vi "EventQueueCluster.vi"() -> ()   [LabVIEW 2017]
uses:
  EventQueueCluster.ctl
  EventMessage.ctl
panel:
  in  "EventQueueCluster":T1
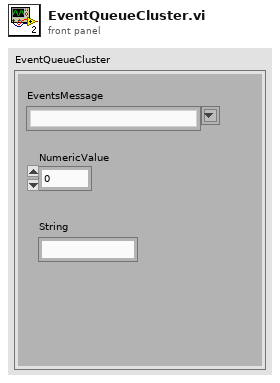
[diagram p1: front panel]
types:
  T1 = typedef "EventQueueCluster.ctl" = cluster{"EventsMessage":T2, "NumericValue":dbl, "String":string}
  T2 = typedef "EventMessage.ctl" = string
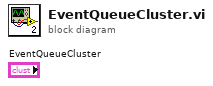
[diagram p0: block diagram]
diagram:
